vi "Start.vi"(8 "error in (no error)":errorcluster, 11 "MQTT_Base in":refnum<class "MQTT_Base.lvclass">) -> (0 "error out":errorcluster, 1 "timed out?":bool, 3 "MQTT_Base out":refnum<class "MQTT_Base.lvclass">)   [LabVIEW 2013, in "MQTT Server.lvlib" / "MQTT_Base.lvclass"]
uses:
  MQTT_Base.lvclass
  MQTT_Base.lvclass/MQTT_Base.ctl
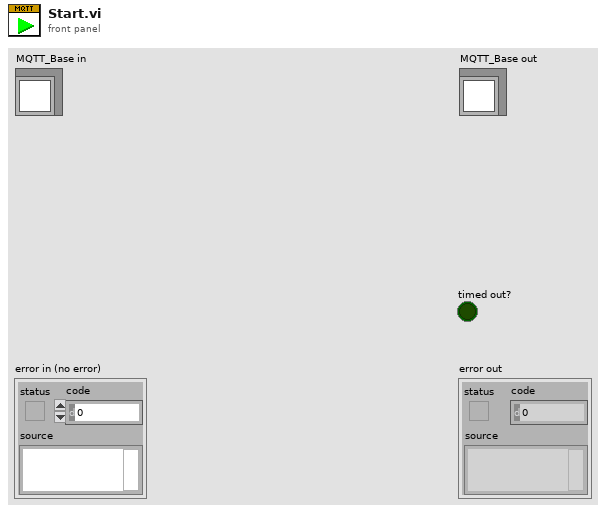
[diagram p1: front panel]
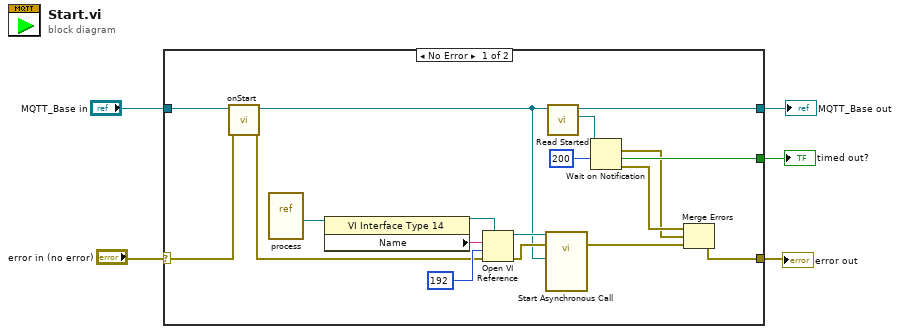
[diagram p0: block diagram]
diagram:
  n1 = case shown="No Error" "error in (no error)" {
    selector: "error in (no error)" -> [w10 w25]
    tunnel: [w12 w25] -> w3
    tunnel: [w7 w24] -> w2
    tunnel: "MQTT_Base in" -> [w11 w24]
    tunnel: [w14 _] -> w1
    frame No Error {
      n2 = call-dynamic "onStart.vi"("error in (no error)"=w10, "MQTT_Base in"=w11) -> ("error out"=w9:errorcluster, "MQTT_Base out"=w6:refnum<class "MQTT_Base.lvclass">)  [unwired: 8 in]
      n3 = vi-ref "process.vi"() -> (w23:refnum<vi>)
      n4 = property class="VI Interface Type 14"(reference=w23) -> (reference out=w21:refnum<vi>, "Name"=w22:string)  [unwired: 1 in, 1 out]
      n5 = Open VI Reference(type specifier VI Refnum (for type only)=w21, vi path=w22, options=192, error in (no error)=w9) -> (vi reference=w20:refnum<vi>, error out=w19:errorcluster)  [unwired: 2 in]
      n6 = call-by-ref "Start Asynchronous Call"(reference=w20, error in=w19, "MQTT_Base in"=w6) -> (error out=w16:errorcluster)  [unwired: 11 in, 1 out]
      n7 = call "Read Started.vi"("MQTT_Base in"=w6) -> ("Started"=w13:refnum<notifier>, "MQTT_Base out"=w7:refnum<class "MQTT_Base.lvclass">)  [unwired: 8 in, 1 out]
      n8 = Wait on Notification(notifier=w13, timeout in ms (-1)=200) -> (notification=w8:errorcluster, timed out?=w14:bool, error out=w15:errorcluster)  [unwired: 2 in, 1 out]
      n9 = Merge Errors(w15, w8, w16) -> (w12:errorcluster)
    }
    frame Error {
    }
  }
  "error out" <- w3
  "MQTT_Base out" <- w2
  "timed out?" <- w1
